vi "set_ram_address.vi"(11 "ram_adress":u16) -> ()   [LabVIEW 2015]
uses:
  <vilib>/rvi/eio/common/nirviEmuTemplateMethod_errors.vi
  <vilib>/eio/EIONode/EIONode.xnode
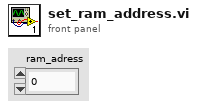
[diagram p1: front panel]
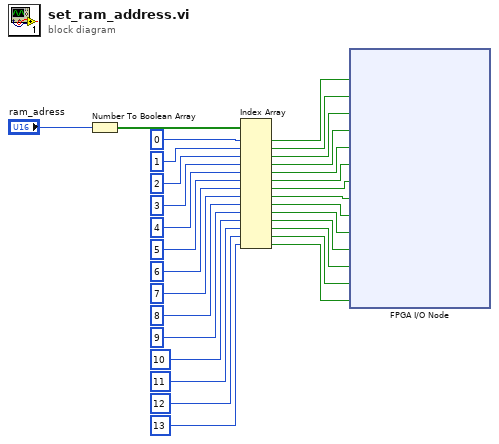
[diagram p0: block diagram]
diagram:
  n1 = Number To Boolean Array(number="ram_adress") -> (Boolean array=w30:bool[])
  n2 = Index Array(array=w30, index #1=0 ("index"), index #2=1 ("index"), index #3=2 ("index"), index #4=3 ("index"), index #5=4 ("index"), index #6=5 ("index"), index #7=6 ("index"), index #8=7 ("index"), index #9=8 ("index"), index #10=9 ("index"), index #11=10 ("index"), index #12=11 ("index"), index #13=12 ("index"), index #14=13 ("index")) -> (element #1=w20:bool, element #2=w19:bool, element #3=w18:bool, element #4=w17:bool, element #5=w16:bool, element #6=w15:bool, element #7=w14:bool, element #8=w13:bool, element #9=w12:bool, element #10=w11:bool, element #11=w10:bool, element #12=w9:bool, element #13=w8:bool, element #14=w7:bool)
  n3 = xnode "FPGA I/O Node"("ram_address[0]"=w20, "ram_address[1]"=w19, "ram_address[2]"=w18, "ram_address[3]"=w17, "ram_address[4]"=w16, "ram_address[5]"=w15, "ram_address[6]"=w14, "ram_address[7]"=w13, "ram_address[8]"=w12, "ram_address[9]"=w11, "ram_address[10]"=w10, "ram_address[11]"=w9, "ram_address[12]"=w8, "ram_address[13]"=w7) -> ()  [unwired: 14 in, 14 out]
